vi "读取增益.vi"(8 "error in":errorcluster) -> (0 "error out":errorcluster, 2 "data":u16, 3 "return":i32)   [LabVIEW 2016]
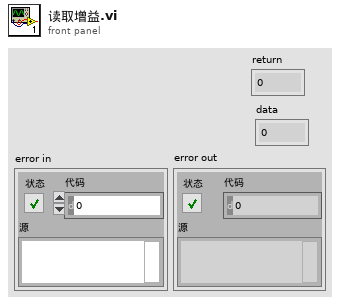
[diagram p1: front panel]
types:
  T1 = cluster{"byCmdType":u8, "bySubCmd":u8, "byParam_h":u8, "byParam_l":u8, "byAddr1_hh":u8, "byAddr1_h":u8, "byAddr1_l":u8, "byAddr1_ll":u8, "byAddr2_hh":u8, "byAddr2_h":u8, "byAddr2_l":u8, "byAddr2_ll":u8, "byLen_hh":u8, "byLen_h":u8, "byLen_l":u8, "byLen_ll":u8}
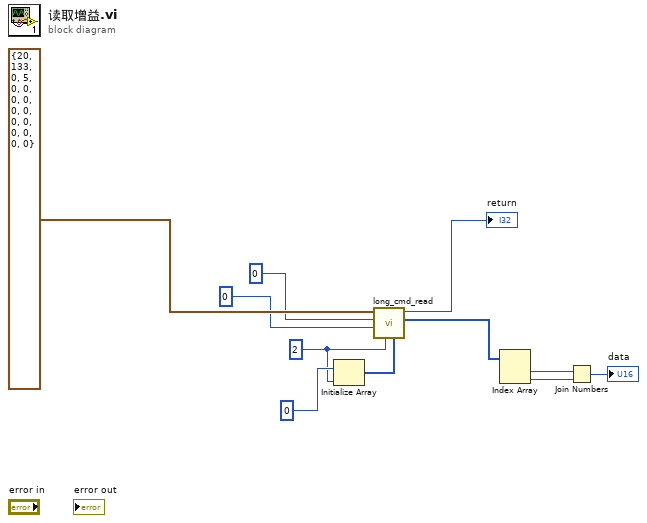
[diagram p0: block diagram]
diagram:
  w1 = u32 2 ("dwLen")
  n1 = Initialize Array(0, w1) -> (w8:i32[])
  n2 = call "long_cmd_read.vi"("data"=w8, "dwLen"=w1, "dwAddr2"=u32 0, "dwAddr1"=u32 0, "vd_cmd_long_header_t"=T1 {"byCmdType"=20, "bySubCmd"=133, "byParam_h"=0, "byParam_l"=5, "byAddr1_hh"=0, "byAddr1_h"=0, "byAddr1_l"=0, "byAddr1_ll"=0, "byAddr2_hh"=0, "byAddr2_h"=0, "byAddr2_l"=0, "byAddr2_ll"=0, "byLen_hh"=0, "byLen_h"=0, "byLen_l"=0, "byLen_ll"=0}) -> ("data out"=w6:u8[], "return"=→"return":i32)  [unwired: 4 in, 1 out]
  n3 = Index Array(array=w6) -> (element #1=w5:u8, element #2=w4:u8)  [unwired: 2 in]
  n4 = Join Numbers(hi=w5, lo=w4) -> ((hi.lo)=→"data":u16)
